vi "Write Buffer.vi"(8 "error in (no error)":errorcluster, 10 "Buffer":string, 11 "Measure in":refnum<class "Measure.lvclass">) -> (0 "error out":errorcluster, 3 "Measure out":refnum<class "Measure.lvclass">)   [LabVIEW 2023, in "HAF.lvlib" / "Measure.lvclass"]
uses:
  Measure.lvclass
  Measure.lvclass/Measure.ctl
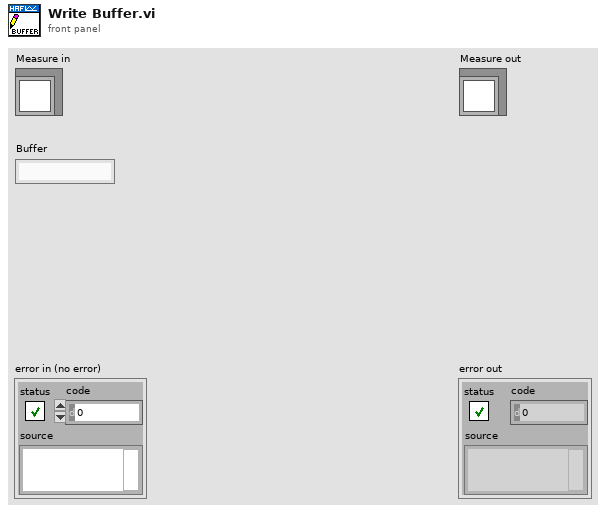
[diagram p1: front panel]
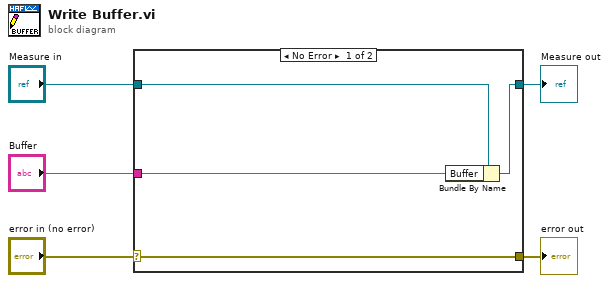
[diagram p0: block diagram]
diagram:
  n1 = case shown="No Error" "error in (no error)" {
    selector: "error in (no error)" -> [w9 w10]
    tunnel: [w9 w10] -> w4
    tunnel: [w7 w11] -> w2
    tunnel: "Measure in" -> [w8 w11]
    tunnel: "Buffer" -> [w6 _]
    frame No Error {
      n2 = Bundle By Name(cluster=w8, "Buffer"=w6) -> (w7:refnum<class "Measure.lvclass">)
    }
    frame Error {
    }
  }
  "error out" <- w4
  "Measure out" <- w2
